vi "shakeServoArduinoNew.vi"(8 "milliseconds to wait":u32=10, 9 "numShakes":i32=3, 10 "shake span":i16=50, 11 "servo id":i32) -> ()   [LabVIEW 2012]
uses:
  GlobalArduinoNew.vi
  <vilib>/LabVIEW Interface for Arduino/LabVIEW Interface for Arduino.lvlib
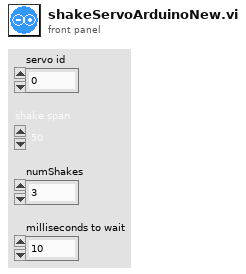
[diagram p1: front panel]
types:
  T1 = typedef "LabVIEW Interface for Arduino.lvlib/Arduino Resource.ctl" = cluster{"VISA resource":refnum<visa-resource-name>, "Board Type":T2, "Connection Type":enum8{"USB / Serial"}, "Bytes Per Packet (15)":u8}
  T2 = typedef "LabVIEW Interface for Arduino.lvlib/Board Type.ctl" = enum16{"Uno", "Dimuelanove w/Atmega 328", "Mega 2560"}
  T3 = typedef "Semaphore RefNum" = refnum<k1>
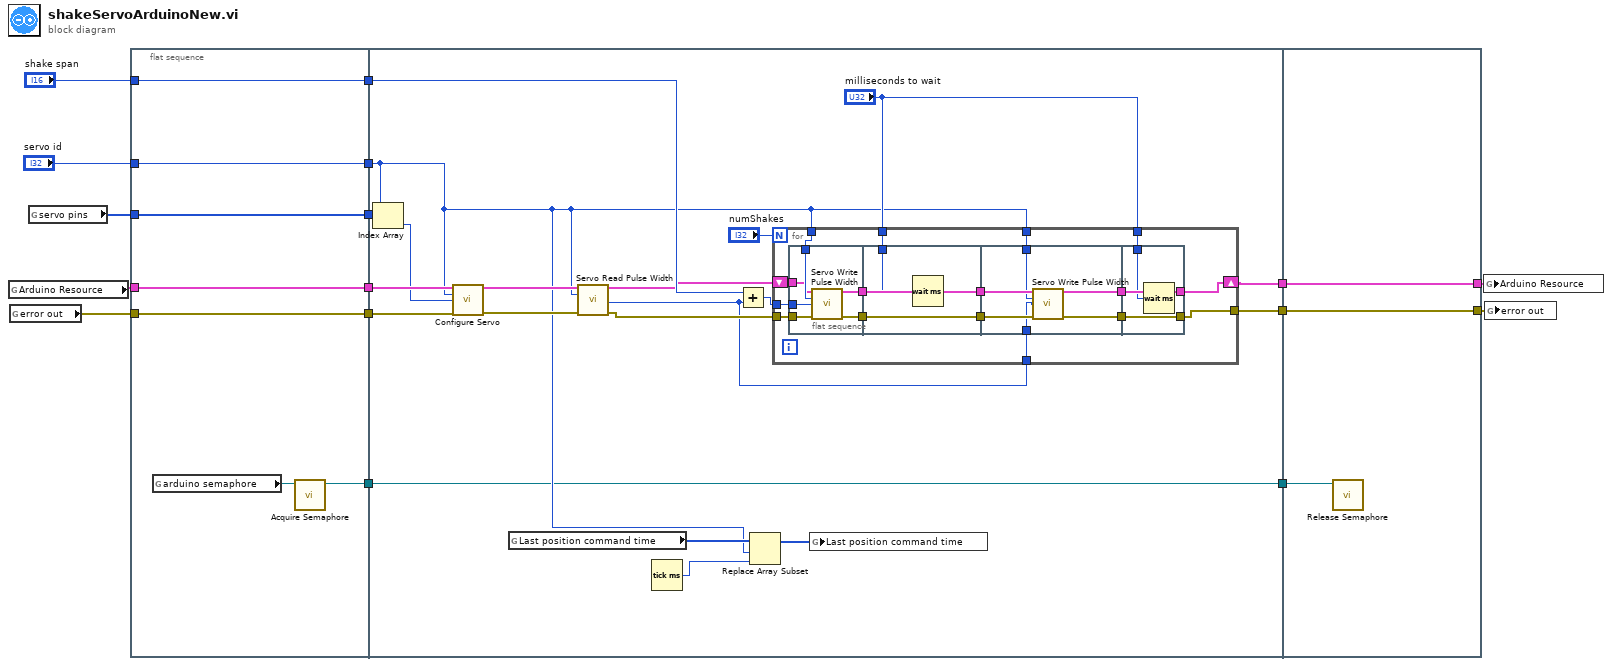
[diagram p0: block diagram]
diagram:
  n1 = global read "GlobalArduinoNew.vi" "Arduino Resource"() -> (w16:T1)
  n2 = global read "GlobalArduinoNew.vi" "error out"() -> (w15:errorcluster)
  n3 = global read "GlobalArduinoNew.vi" "servo pins"() -> (w14:u8[])
  n4 = flat-sequence {
    tunnel: "servo id" -> [w19]
    tunnel: "shake span" -> [w20]
    tunnel: w14 -> [w21]
    tunnel: w15 -> [w22]
    tunnel: w16 -> [w23]
    tunnel: [w23] -> w9
    tunnel: [w22] -> w8
    tunnel: [w21] -> w7
    tunnel: [w20] -> w6
    tunnel: [w19] -> w5
    tunnel: [w17] -> w2
    tunnel: w9 -> [w43]
    tunnel: w8 -> [w42]
    tunnel: w7 -> [w40]
    tunnel: w6 -> [w33]
    tunnel: w5 -> [w25]
    tunnel: [w27] -> w4
    tunnel: [w26] -> w3
    tunnel: w2 -> [w24]
    tunnel: [w24] -> w1
    tunnel: [w79] -> w11
    tunnel: [w80] -> w12
    tunnel: w4 -> [w80]
    tunnel: w3 -> [w79]
    tunnel: w1 -> [w78]
    frame #0 {
      n5 = global read "GlobalArduinoNew.vi" "arduino semaphore"() -> (w18:T3)
      n6 = call <vilib>:"Acquire Semaphore.vi"("semaphore"=w18) -> ("semaphore out"=w17:T3)  [unwired: 4 in, 2 out]
    }
    frame #1 {
      n7 = Index Array(array=w40, index=w25) -> (element=w41:u8)
      n8 = call <vilib>:"Configure Servo.vi"("Arduino Resource"=w43, "Servo Number (0)"=w25, "DIO Pin (2)"=w41, "error in"=w42) -> ("Arduino Resource"=w36:T1, "error out"=w35:errorcluster)  [unwired: 10 in]
      n9 = global read "GlobalArduinoNew.vi" "Last position command time"() -> (w38:u64[])
      n10 = call <vilib>:"Servo Read Pulse Width.vi"("Arduino Resource"=w36, "Servo Number"=w25, "error in"=w35) -> ("Arduino Resource"=w30:T1, "Pulse Width in uS"=w28:u16, "error out"=w31:errorcluster)  [unwired: 10 in]
      n11 = Tick Count (ms)() -> (millisecond timer value=w37:u32)
      n12 = Add(x=w33, y=w28) -> (x+y=w32:u16)
      n13 = Replace Array Subset(array=w38, new element=w37, index=w25) -> (w39:u64[])
      n14 = for {
        N: "numShakes" -> [_]
        tunnel: w32 -> [w59]
        tunnel: w25 -> [w58]
        tunnel: w31 -> [w57]
        shift-right: [w45] -> w27
        shift-left: w30 -> [w56]
        tunnel: "milliseconds to wait" -> [w49]
        tunnel: "milliseconds to wait" -> [w48]
        tunnel: w25 -> [w47]
        tunnel: w28 -> [w46]
        tunnel: [w44] -> w26
        n15 = flat-sequence {
          tunnel: w59 -> [w65]
          tunnel: w58 -> [w64]
          tunnel: w57 -> [w63]
          tunnel: w56 -> [w62]
          tunnel: [w61] -> w55
          tunnel: [w60] -> w54
          tunnel: w55 -> [w68]
          tunnel: w54 -> [w67]
          tunnel: [w68] -> w53
          tunnel: [w67] -> w52
          tunnel: w49 -> [w66]
          tunnel: w53 -> [w74]
          tunnel: w52 -> [w72]
          tunnel: [w73] -> w51
          tunnel: [w71] -> w50
          tunnel: w47 -> [w70]
          tunnel: w46 -> [w69]
          tunnel: [w76] -> w44
          tunnel: [w77] -> w45
          tunnel: w51 -> [w77]
          tunnel: w50 -> [w76]
          tunnel: w48 -> [w75]
          frame #0 {
            n16 = call <vilib>:"Servo Write Pulse Width.vi"("Arduino Resource"=w62, "Servo Number"=w64, "Pulse Width in uS"=w65, "error in"=w63) -> ("Arduino Resource"=w61:T1, "error out"=w60:errorcluster)  [unwired: 10 in]
          }
          frame #1 {
            n17 = Wait (ms)(milliseconds to wait=w66) -> ()  [unwired: 1 out]
          }
          frame #2 {
            n18 = call <vilib>:"Servo Write Pulse Width.vi"("Arduino Resource"=w74, "Servo Number"=w70, "Pulse Width in uS"=w69, "error in"=w72) -> ("Arduino Resource"=w73:T1, "error out"=w71:errorcluster)  [unwired: 10 in]
          }
          frame #3 {
            n19 = Wait (ms)(milliseconds to wait=w75) -> ()  [unwired: 1 out]
          }
        }
      }
      n20 = global write "GlobalArduinoNew.vi" "Last position command time"(w39) -> ()
    }
    frame #2 {
      n21 = call <vilib>:"Release Semaphore.vi"("semaphore"=w78) -> ()  [unwired: 5 in, 2 out]
    }
  }
  n22 = global write "GlobalArduinoNew.vi" "Arduino Resource"(w12) -> ()
  n23 = global write "GlobalArduinoNew.vi" "error out"(w11) -> ()
